vi "hyperextension_detection.vi"() -> ()   [LabVIEW 2025]
uses:
  <vilib>/ptbypt/NI_PtbyPt.lvlib
panel:
  out "Hyperextension?":bool
  out "Direction":i32
  in  "Hyperextension Angle Limit (degrees)":dbl=60.0
  out "Coerced Speed":dbl
  in  "Motor Speed Limit (rpm)":dbl=13.0
  in  "motor radius":dbl=0.2
  out "Known Speed":dbl
  out "Acceleration":dbl(graph)
  out "Relative Position":dbl(graph)
  out "Speed":dbl(graph)
  in  "Speed Selection (simulation only)":i32=2
  out "Force":dbl(graph)
  out "D":bool
  out "C":bool
  out "B":bool
  out "A":bool
  out "dT":dbl
  in  "stop":bool
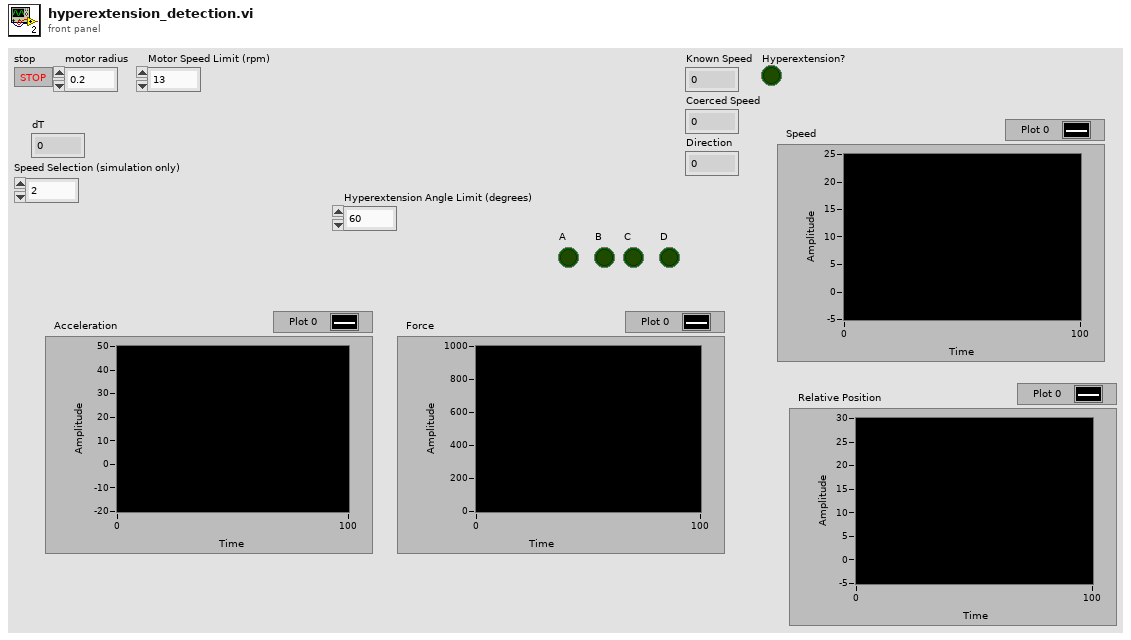
[diagram p1: front panel]
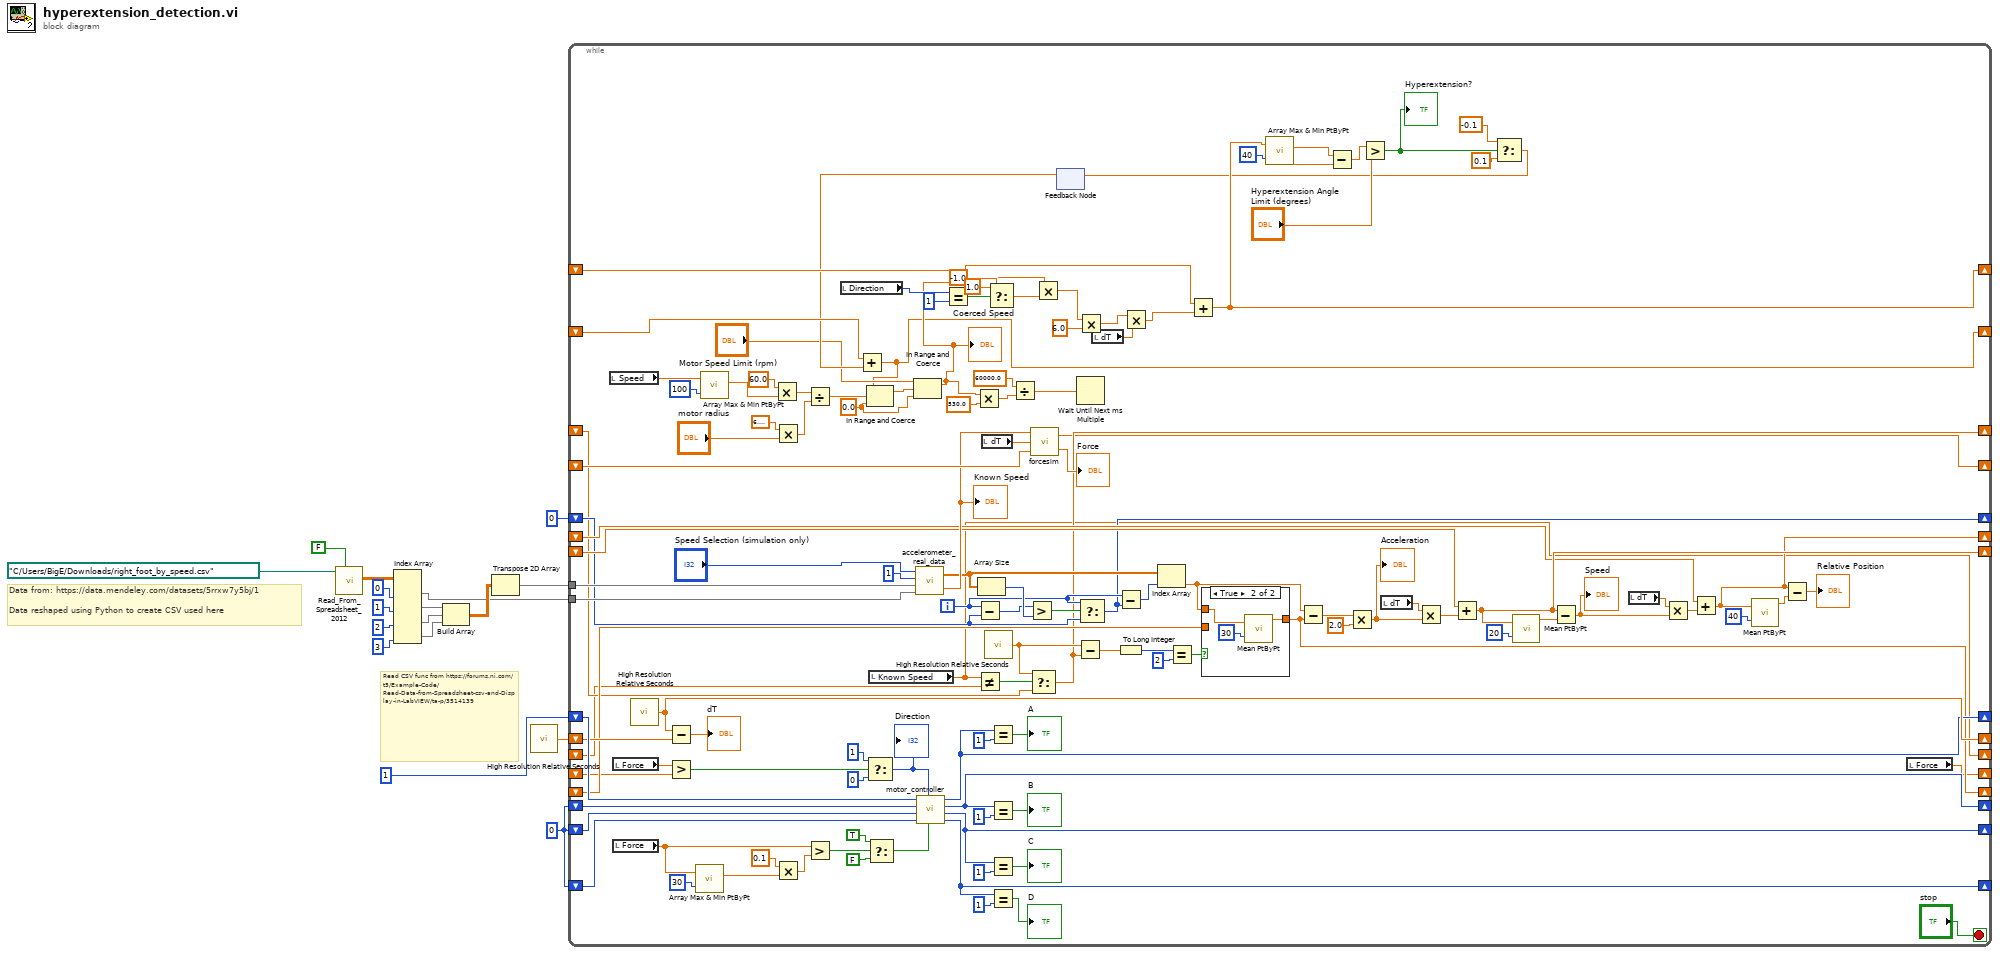
[diagram p0: block diagram]
diagram:
  w15 = 0
  # "Data from: https://data.mendeley.com/datasets/5rrxw7y5bj/1\n\nData reshaped using Python to create CSV used here"
  # "Read CSV func from https://forums.ni.com/t5/Example-Code/Read-Data-from-Spreadsheet-csv-and-Display-in-LabVIEW/ta-p/3514139"
  n1 = call "Read_From_Spreadsheet_2012.vi"("My File has Row Headers"=FALSE, "Spreadsheet path (.csv)"=path "C:/Users/BigE/Downloads/right_foot_by_speed.csv") -> ("Data Dsiplay"=w10:dbl[][])  [unwired: 8 in, 1 out]
  n2 = Index Array(array=w10, index (col) #1=0 ("disabled index (col)"), index (col) #2=1 ("disabled index (col)"), index (col) #3=2 ("disabled index (col)"), index (col) #4=3 ("disabled index (col)")) -> (element #1=w3:dbl[], element #2=w11:dbl[], element #3=w12:dbl[], element #4=w13:dbl[])  [unwired: 4 in]
  n3 = Build Array(w11, w12, w13) -> (w14:dbl[][])
  n4 = Transpose 2D Array(2D array=w14) -> (transposed array=w2:dbl[][])
  n5 = call <vilib>:"High Resolution Relative Seconds.vi"() -> ("relative seconds"=w17:dbl)
  n6 = while {
    shift-right: [w132] -> _
    shift-left: 1 -> [w141]
    shift-right: [w128] -> _
    shift-left: w15 -> [w140]
    shift-right: [w127] -> _
    shift-left: w15 -> [w139]
    shift-right: [w126] -> _
    shift-left: w15 -> [w138]
    shift-right: [w67] -> _
    shift-left: _ -> [w137]
    shift-right: [w135] -> _
    shift-left: w17 -> [w136]
    tunnel: w3 -> [w117]
    tunnel: w2 -> [w115]
    shift-right: [w108] -> _
    shift-left: _ -> [w106]
    shift-right: [w107] -> _
    shift-left: _ -> [w105]
    shift-right: [w95] -> _
    shift-left: 0 -> [w97]
    shift-right: [w92] -> _
    shift-left: _ -> [w93]
    shift-right: [w83] -> _
    shift-left: _ -> [w84]
    shift-right: [w81] -> _
    shift-left: _ -> [w80]
    shift-right: [w66] -> _
    shift-left: _ -> [w64]
    shift-right: [w33] -> _
    shift-left: _ -> [w42]
    shift-right: [w18] -> _
    shift-left: _ -> [w22]
    i -> [w96]
    stop <- "stop" stop-if-true
    w25 = 0.0 ("lower limit")
    n7 = local read "Speed"() -> (w58:dbl)
    n8 = local read "Force"() -> (w65:dbl)
    n9 = local read "Force"() -> (w63:dbl)
    n10 = call <vilib>:"High Resolution Relative Seconds.vi"() -> ("relative seconds"=w135:dbl)
    n11 = Subtract(x=w135, y=w136) -> (x-y=→"dT":dbl)
    n12 = Greater?(x=w65, y=w64) -> (0:w72:bool)
    n13 = call <vilib>:"Array Max & Min PtByPt.vi"("input data point"=w63, "sample length"=30) -> ("max value"=w68:dbl)  [unwired: 1 in, 4 out]
    n14 = call <vilib>:"Array Max & Min PtByPt.vi"("input data point"=w58, "sample length"=100) -> ("max value"=w56:dbl)  [unwired: 1 in, 4 out]
    n15 = Multiply(x=60.0, y=w56) -> (x*y=w52:dbl)
    n16 = Multiply(x=6.283185307179586, y="motor radius") -> (x*y=w53:dbl)
    n17 = Multiply(x=0.1, y=w68) -> (x*y=w75:dbl)
    n18 = Divide(x=w52, y=w53) -> (x/y=w51:dbl)
    n19 = Greater?(x=w63, y=w75) -> (0:w74:bool)
    n20 = local read "Direction"() -> (w39:i32)
    n21 = Select(t=1, s=w72, f=0) -> (s? t:f=w60:i32)
    "Direction" <- w60
    n22 = Select(t=TRUE, s=w74, f=FALSE) -> (s? t:f=w61:bool)
    n23 = local read "Known Speed"() -> (w81:dbl)
    n24 = call "accelerometer_real_data.vi"("speed subarray"=w117, "transposed array"=w115, "x,y,z?"=1, "Speed Index"="Speed Selection (simulation only)") -> ("Speed"=w118:dbl, "Accleration Array"=w101:dbl[])
    "Known Speed" <- w118
    n25 = call "motor_controller.vi"("On/Off"=w61, "U"=w60, "D Prev"=w138, "C Prev"=w139, "B Prev"=w140, "A Prev"=w141) -> ("D Curr"=w126:i32, "C Curr"=w127:i32, "B Curr"=w128:i32, "A Curr"=w132:i32)
    n26 = Equal?(x=w39, y=1) -> (x = y?=w40:bool)
    n27 = Subtract(x=w96, y=w97) -> (x-y=w99:i32)
    n28 = Not Equal?(x=w81, y=w80) -> (x != y?=w82:bool)
    n29 = Array Size(array=w101) -> (size(s)=w100:i32)
    n30 = local read "dT"() -> (w134:dbl)
    n31 = call <vilib>:"High Resolution Relative Seconds.vi"() -> ("relative seconds"=w85:dbl)
    n32 = Select(t=1.0, s=w40, f=-1.0) -> (s? t:f=w41:dbl)
    n33 = Equal?(x=w132, y=1) -> (x = y?=→"A":bool)
    n34 = Equal?(x=w128, y=1) -> (x = y?=→"B":bool)
    n35 = Equal?(x=w127, y=1) -> (x = y?=→"C":bool)
    n36 = Equal?(x=w126, y=1) -> (x = y?=→"D":bool)
    n37 = Greater?(x=w99, y=w100) -> (0:w98:bool)
    n38 = Select(t=w85, s=w82, f=w84) -> (s? t:f=w83:dbl)
    n39 = call "forcesim.vi"("Phase"=w137, "dT"=w134, "Speed"=w118) -> ("Force"=→"Force":dbl, "Phase Out"=w67:dbl)
    n40 = feedback #1() -> (w20:dbl)  [unwired: 1 in]
    n41 = Add(x=w22, y=w20) -> (x+y=w18:dbl)
    n42 = In Range and Coerce(upper limit=w18, x=w51, lower limit=w25) -> (coerced(x)=w26:dbl)  [unwired: 1 out]
    n43 = In Range and Coerce(upper limit="Motor Speed Limit (rpm)", x=w26, lower limit=w25) -> (coerced(x)=w24:dbl)  [unwired: 1 out]
    "Coerced Speed" <- w24
    n44 = Multiply(x=w24, y=530.0) -> (x*y=w49:dbl)
    n45 = Divide(x=60000.0, y=w49) -> (x/y=w47:dbl)
    n46 = Multiply(x=w24, y=w41) -> (x*y=w35:dbl)
    n47 = Wait Until Next ms Multiple(millisecond multiple=w47) -> ()  [unwired: 1 out]
    n48 = Subtract(x=w85, y=w83) -> (x-y=w88:dbl)
    n49 = Multiply(x=w35, y=6.0) -> (x*y=w44:dbl)
    n50 = Select(t=w96, s=w98, f=w97) -> (s? t:f=w95:i32)
    n51 = local read "dT"() -> (w45:dbl)
    n52 = Subtract(x=w96, y=w95) -> (x-y=w94:i32)
    n53 = To Long Integer(number=w88) -> (32bit integer=w89:i32)
    n54 = Multiply(x=w44, y=w45) -> (x*y=w43:dbl)
    n55 = Index Array(array=w101, index=w94) -> (element=w91:dbl)
    n56 = Equal?(x=w89, y=2) -> (x = y?=w86:bool)
    n57 = Add(x=w42, y=w43) -> (x+y=w33:dbl)
    n58 = case shown="True" w86 {
      tunnel: w91 -> [_ w145]
      tunnel: [w143 w144] -> w92
      tunnel: w93 -> [w143 _]
      frame False {
      }
      frame True {
        n59 = call <vilib>:"Mean PtByPt.vi"("x"=w145, "sample length"=30) -> ("mean"=w144:dbl)  [unwired: 2 in, 1 out]
      }
    }
    n60 = call <vilib>:"Array Max & Min PtByPt.vi"("input data point"=w33, "sample length"=40) -> ("max value"=w32:dbl, "min value"=w31:dbl)  [unwired: 1 in, 3 out]
    n61 = Subtract(x=w91, y=w92) -> (x-y=w90:dbl)
    n62 = Subtract(x=w32, y=w31) -> (x-y=w30:dbl)
    n63 = Multiply(x=w90, y=2.0) -> (x*y=w78:dbl)
    "Acceleration" <- w78
    n64 = Greater?(x=w30, y="Hyperextension Angle Limit (degrees)") -> (0:w28:bool)
    "Hyperextension?" <- w28
    n65 = local read "dT"() -> (w104:dbl)
    n66 = Multiply(x=w104, y=w78) -> (x*y=w109:dbl)
    n67 = Add(x=w106, y=w109) -> (x+y=w108:dbl)
    n68 = Select(t=-0.1, s=w28, f=0.1 ("t")) -> (s? t:f=w21:dbl)
    n69 = feedback-in #1(w21) -> ()
    n70 = call <vilib>:"Mean PtByPt.vi"("x"=w108, "sample length"=20) -> ("mean"=w113:dbl)  [unwired: 2 in, 1 out]
    n71 = Subtract(x=w108, y=w113) -> (x-y=w79:dbl)
    "Speed" <- w79
    n72 = local read "dT"() -> (w103:dbl)
    n73 = Multiply(x=w103, y=w79) -> (x*y=w110:dbl)
    n74 = Add(x=w105, y=w110) -> (x+y=w107:dbl)
    n75 = call <vilib>:"Mean PtByPt.vi"("x"=w107, "sample length"=40) -> ("mean"=w111:dbl)  [unwired: 2 in, 1 out]
    n76 = Subtract(x=w107, y=w111) -> (x-y=→"Relative Position":dbl)
    n77 = local read "Force"() -> (w66:dbl)
  }
